vi "Write Value.vi"(8 "error in (no error)":errorcluster, 10 "Value":i64, 11 "sfixed64 in":refnum<class "sfixed64.lvclass">) -> (0 "error out":errorcluster, 3 "sfixed64 out":refnum<class "sfixed64.lvclass">)   [LabVIEW 2020, in "Protobuf RAW.lvlib" / "sfixed64.lvclass"]
uses:
  sfixed64.lvclass
  sfixed64.lvclass/sfixed64.ctl
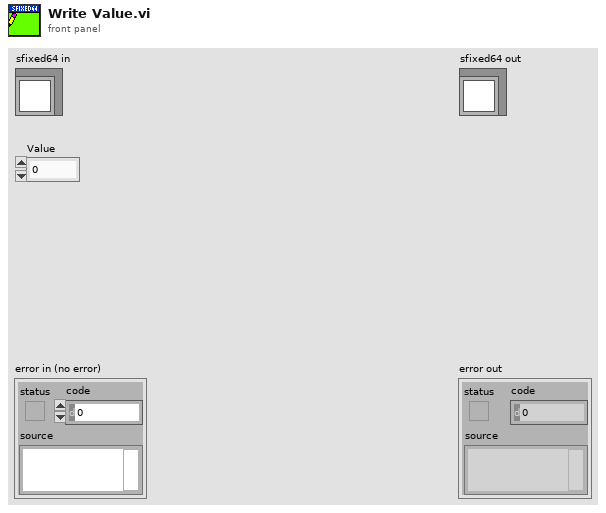
[diagram p1: front panel]
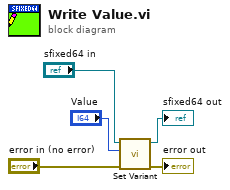
[diagram p0: block diagram]
diagram:
  n1 = call-dynamic "Set Variant.vi"("error in (no error)"="error in (no error)", "Value"="Value", "Proto Type Common in"="sfixed64 in") -> ("error out"=→"error out":errorcluster, "Proto Type Common out"=→"sfixed64 out":refnum<class "sfixed64.lvclass">)  [unwired: 7 in]
